vi "Setup webcam (SubVI).vi"(8 "error in (no error)":errorcluster) -> (0 "error out":errorcluster, 2 "New Image":T2, 3 "Refnum out":T1)   [LabVIEW 2014]
uses:
  <vilib>/vision/Image Controls.llb/IMAQ Image.ctl
  <vilib>/userdefined/High Color/IMAQdx.ctl
  <vilib>/vision/driver/NI_Vision_Acquisition_Software.lvlib
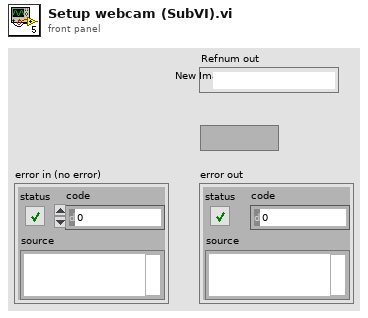
[diagram p1: front panel]
types:
  T1 = typedef "IMAQdx.ctl" = refnum<k21>
  T2 = typedef "IMAQ Image.ctl" = refnum<image>
  T3 = typedef "Image Type" = u32
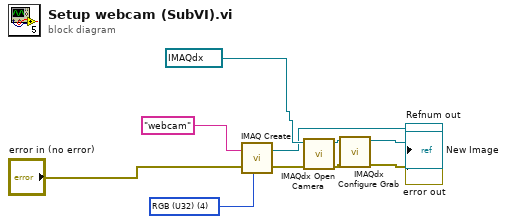
[diagram p0: block diagram]
diagram:
  w5 = T3 4 items=["Grayscale (U8)", "Grayscale (I16)", "Grayscale (SGL)", "Complex (CSG)", "RGB (U32)", "HSL (U32)", "RGB (U64)", "Grayscale (U16)"] ("Image Type")
  n1 = call "IMAQ Create"("Image Name"="webcam", "Image Type"=w5, "error in (no error)"="error in (no error)") -> ("New Image"=→"New Image":T2, "error out"=w8:errorcluster)  [unwired: 2 in]
  n2 = call <vilib>:"IMAQdx Open Camera.vi"("error in"=w8, "Session In"=T1 "cam0") -> ("error out"=w4:errorcluster, "Session Out"=w3:T1)  [unwired: 8 in]
  n3 = call <vilib>:"IMAQdx Configure Grab.vi"("error in"=w4, "Session In"=w3) -> ("error out"=→"error out":errorcluster, "Session Out"=→"Refnum out":T1)  [unwired: 8 in]
